vi "test final.vi"(1 "Array":dbl[][](array[numeric]), 2 "2p":string, 3 "1p":string) -> ()   [LabVIEW 2014]
panel:
  in  "finish":bool
  in  "onemore":bool
  out "Array 2":dbl[][](array[numeric])
  out "2p 2":string
  out "1p 2":string
  # "分數"
  # "害死青蛙數"
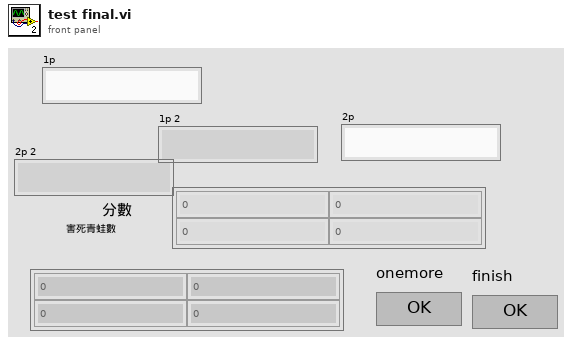
[diagram p1: front panel]
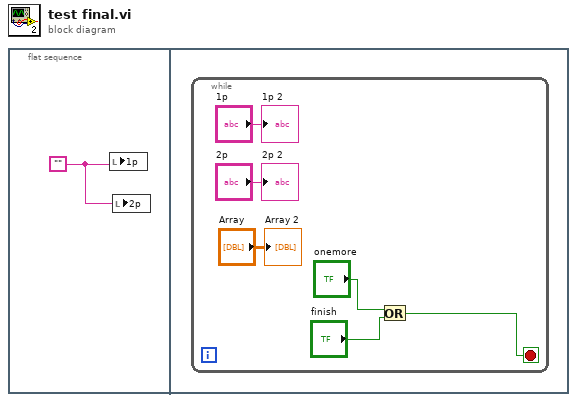
[diagram p0: block diagram]
diagram:
  n1 = flat-sequence {
    frame #0 {
      w1 = ""
      n2 = local write "1p"(w1) -> ()
      n3 = local write "2p"(w1) -> ()
    }
    frame #1 {
      n4 = while {
        stop <- w2 stop-if-true
        n5 = Or(x="onemore", y="finish") -> (x .or. y?=w2:bool)
        "1p 2" <- "1p"
        "2p 2" <- "2p"
        "Array 2" <- "Array"
      }
    }
  }
